vi "String to Null.vi"(11 "String":string) -> (3 "s? t:f":string)   [LabVIEW 2021, in "DataBase_SQL.lvclass"]
doc: "if string is empty ,input NULL."
uses:
  <userlib>/John_Lib/DataBase/DataBase_SQL/DataBase_SQL.lvclass
  <userlib>/John_Lib/DataBase/DataBase_SQL/DataBase_SQL.lvclass/DataBase_SQL.ctl
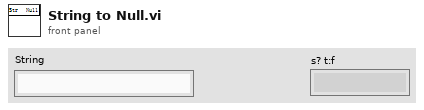
[diagram p1: front panel]
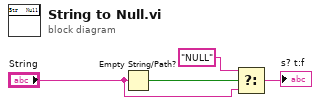
[diagram p0: block diagram]
diagram:
  n1 = Empty String/Path?(string/path="String") -> (empty?=w4:bool)
  n2 = Select(t="NULL", s=w4, f="String") -> (s? t:f=→"s? t:f":string)
